vi "pp3_log_sessionParameters.vi"(10 "queue in":refnum<queue>, 11 "Session parameters":T1={"Log File Directory Root"=path "C:/test", "Habit tr0 (s)"=180, "ITI max\n(s)"=25, "ITI min\n(s)"=15, "Tone repeat (ms)"=0, "Jump time\n(s)"=4, "Subject Name"="SPP030", "Run"=FALSE, "Start trial"=0, "Stay \n(s)"=5, "Log File Directory"=path "", "Shock \ndur (s)"=6, "Pre click \n(V)"=1.0, "Click\ndel (s)"=6.0} {"Click\ndel (s)" min=0.0 step=1.0; "Pre click \n(V)" min=0.0 step=1.0; "Shock \ndur (s)" min=0 step=1; "Stay \n(s)" min=0 step=1; "Start trial" step=1; "Jump time\n(s)" min=0 step=1; "Tone repeat (ms)" min=0 step=1; "ITI min\n(s)" min=0 step=1; "ITI max\n(s)" min=0 step=1; "Habit tr0 (s)" min=0 step=1}) -> (2 "queue out":refnum<queue>)   [LabVIEW 2013]
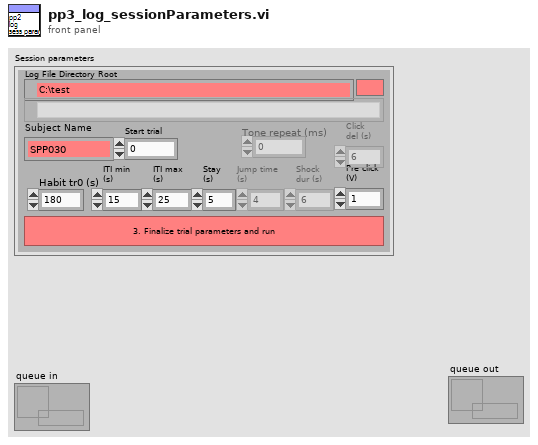
[diagram p1: front panel]
types:
  T1 = cluster{"Log File Directory Root":path, "Habit tr0 (s)":i32, "ITI max\n(s)":i32, "ITI min\n(s)":i32, "Tone repeat (ms)":i32, "Jump time\n(s)":i32, "Subject Name":string, "Run":bool, "Start trial":u16, "Stay \n(s)":i32, "Log File Directory":path, "Shock \ndur (s)":i32, "Pre click \n(V)":dbl, "Click\ndel (s)":dbl}
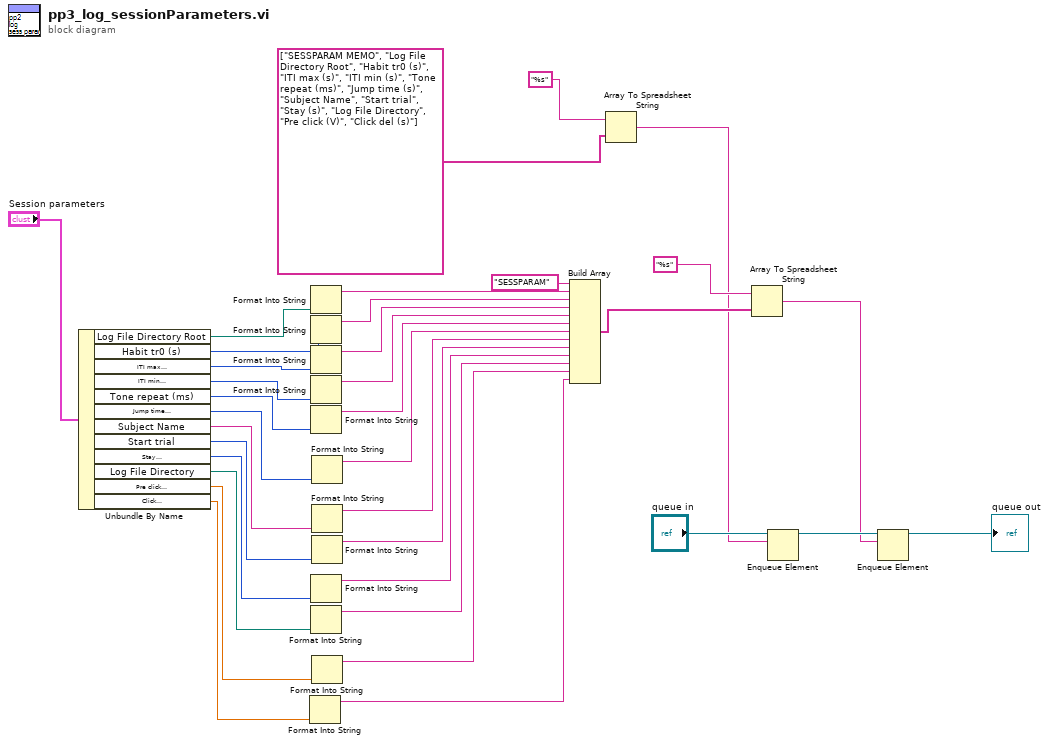
[diagram p0: block diagram]
diagram:
  n1 = Unbundle By Name("Session parameters") -> ("Log File Directory Root"=w35:path, "Habit tr0 (s)"=w32:i32, "ITI max\n(s)"=w31:i32, "ITI min\n(s)"=w30:i32, "Tone repeat (ms)"=w29:i32, "Jump time\n(s)"=w28:i32, "Subject Name"=w22:string, "Start trial"=w21:u16, "Stay \n(s)"=w20:i32, "Log File Directory"=w19:path, "Pre click \n(V)"=w18:dbl, "Click\ndel (s)"=w9:dbl)
  n2 = Format Into String(w9) -> (resulting string=w8:string)  [unwired: 3 in, 1 out]
  n3 = Format Into String(w35) -> (resulting string=w34:string)  [unwired: 3 in, 1 out]
  n4 = Format Into String(w32) -> (resulting string=w27:string)  [unwired: 3 in, 1 out]
  n5 = Format Into String(w31) -> (resulting string=w26:string)  [unwired: 3 in, 1 out]
  n6 = Format Into String(w30) -> (resulting string=w25:string)  [unwired: 3 in, 1 out]
  n7 = Format Into String(w29) -> (resulting string=w24:string)  [unwired: 3 in, 1 out]
  n8 = Format Into String(w20) -> (resulting string=w15:string)  [unwired: 3 in, 1 out]
  n9 = Format Into String(w19) -> (resulting string=w14:string)  [unwired: 3 in, 1 out]
  n10 = Format Into String(w28) -> (resulting string=w23:string)  [unwired: 3 in, 1 out]
  n11 = Format Into String(w22) -> (resulting string=w17:string)  [unwired: 3 in, 1 out]
  n12 = Format Into String(w21) -> (resulting string=w16:string)  [unwired: 3 in, 1 out]
  n13 = Format Into String(w18) -> (resulting string=w13:string)  [unwired: 3 in, 1 out]
  n14 = Build Array("SESSPARAM" ("element"), w34, w27, w26, w25, w24, w23, w17, w16, w15, w14, w13, w8) -> (w11:string[])
  n15 = Array To Spreadsheet String(array=string[] ["SESSPARAM MEMO", "Log File Directory Root", "Habit tr0 (s)", "ITI max (s)", "ITI min (s)", "Tone repeat (ms)", "Jump time (s)", "Subject Name", "Start trial", "Stay (s)", "Log File Directory", "Pre click (V)", "Click del (s)"], 3:"%s" ("format string")) -> (spreadsheet string=w2:string)  [unwired: 1 in]
  n16 = Array To Spreadsheet String(array=w11, 3:"%s" ("format string")) -> (spreadsheet string=w1:string)  [unwired: 1 in]
  n17 = Enqueue Element(queue="queue in", element=w2) -> (queue out=w4:refnum<queue>)  [unwired: 2 in, 2 out]
  n18 = Enqueue Element(queue=w4, element=w1) -> (queue out=→"queue out":refnum<queue>)  [unwired: 2 in, 2 out]
